vi "AverageAndLog.vi"(5 "error in (no error)":errorcluster) -> (19 "error out":errorcluster)   [LabVIEW 2014, in "IndoorData.lvclass"]
uses:
  IndoorData.lvclass
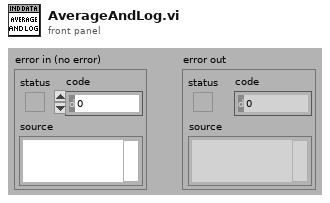
[diagram p1: front panel]
types:
  T1 = enum16{"open", "replace", "create", "open or create", "replace or create", "replace or create with confirmation"}
  T2 = typedef "IndoorData.lvclass/ObjectAttributes.ctl" = cluster{"DebugData":T3, "Actual":T4, "BufferedReadings":T5, "AVGReadings":T5, "LogFolder":path, "FirstLog?":bool, "MinMaxFile":path}
  T3 = typedef "IndoorData.lvclass/DebugData.ctl" = cluster{"Rev":string, "Location":string, "LoopIdx":i32, "PiCoreTemp":dbl, "Error":errorcluster}
  T4 = typedef "IndoorData.lvclass/ActualValues.ctl" = cluster{"Time":dbl, "Temp":dbl, "RH":dbl}
  T5 = typedef "IndoorData.lvclass/BufferedReadings.ctl" = cluster{"Time":dbl[], "Temp":dbl[], "RH":dbl[]}
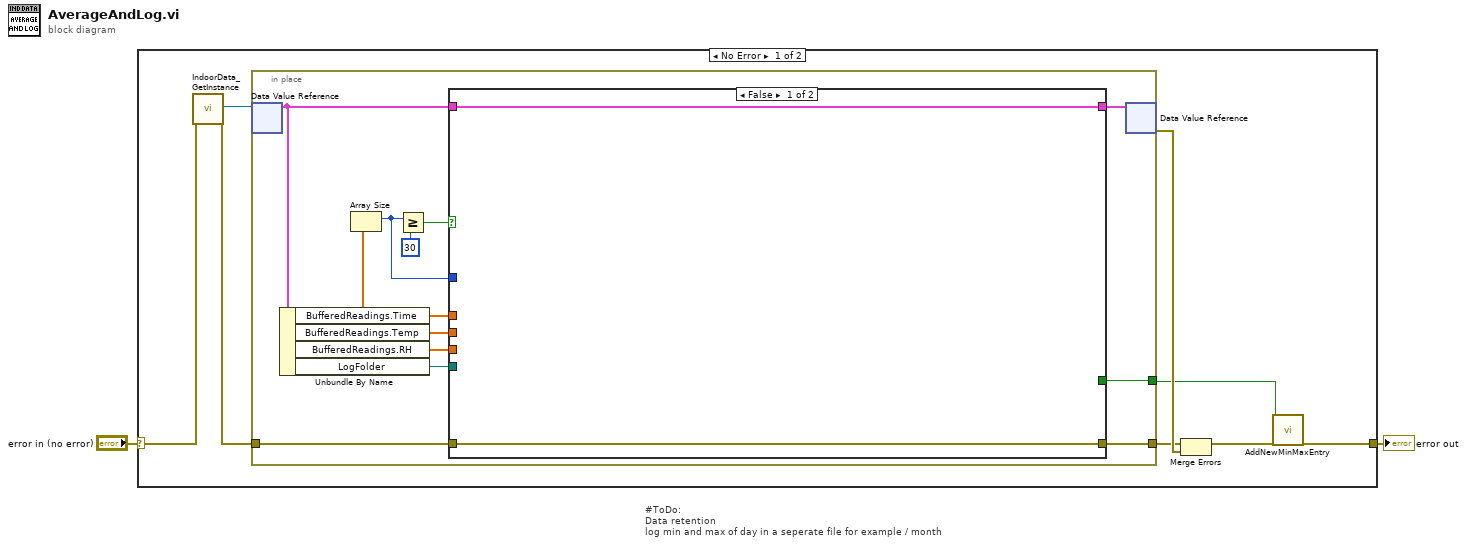
[diagram p0: block diagram]
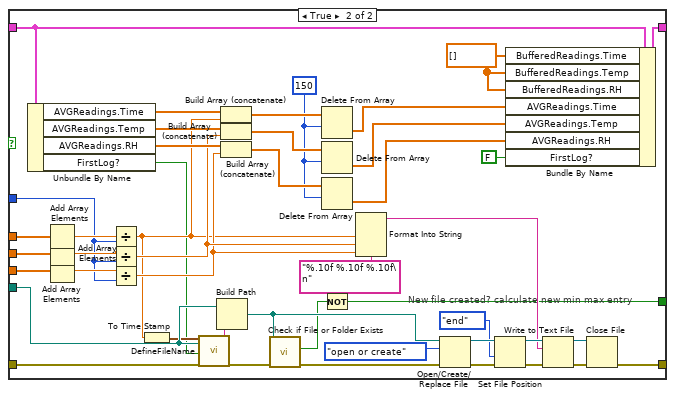
[diagram p2: hidden frame]
diagram:
  # "#ToDo:\nData retention\nlog min and max of day in a seperate file for example / month"
  n1 = case shown="No Error" "error in (no error)" {
    selector: "error in (no error)" -> [w6 w70]
    tunnel: [w4 w70] -> w1
    frame No Error {
      n2 = call "IndoorData_GetInstance.vi"("error in (no error)"=w6) -> ("DVRRefOut"=w9:refnum<data-value>, "error out"=w8:errorcluster)  [unwired: 14 in, 3 out]
      n3 = in-place {
        in-place-border: w8 -> [w17]
        in-place-border: [w18] -> w7
        in-place-border: [w11] -> w3
        n4 = in-place-dvr #1(w9) -> (w21:T2)  [unwired: 1 out]
        n5 = Unbundle By Name(w21) -> ("BufferedReadings.Time"=w16:dbl[], "BufferedReadings.Temp"=w15:dbl[], "BufferedReadings.RH"=w14:dbl[], "LogFolder"=w12:path)
        n6 = Array Size(array=w16) -> (size(s)=w13:i32)
        n7 = Greater Or Equal?(x=w13, y=30) -> (x >= y?=w19:bool)
        n8 = case shown="False" w19 {
          tunnel: [w24 w69] -> w22
          tunnel: w21 -> [w24 w60]
          tunnel: [w23 w37] -> w18
          tunnel: w17 -> [w23 w46]
          tunnel: w16 -> [_ w68]
          tunnel: w15 -> [_ w67]
          tunnel: w14 -> [_ w66]
          tunnel: w13 -> [_ w62]
          tunnel: w12 -> [_ w34]
          tunnel: [_ w25] -> w11
          frame False {
          }
          frame True {
            w53 = 150 ("length")
            w61 = dbl[] [] ("BufferedReadings.Time")
            # "New file created? calculate new min max entry"
            n9 = Unbundle By Name(w60) -> ("AVGReadings.Time"=w59:dbl[], "AVGReadings.Temp"=w58:dbl[], "AVGReadings.RH"=w57:dbl[], "FirstLog?"=w30:bool)
            n10 = Add Array Elements(numeric array=w68) -> (sum=w65:dbl)
            n11 = Add Array Elements(numeric array=w67) -> (sum=w64:dbl)
            n12 = Add Array Elements(numeric array=w66) -> (sum=w63:dbl)
            n13 = Divide(x=w65, y=w62) -> (x/y=w33:dbl)
            n14 = Divide(x=w64, y=w62) -> (x/y=w48:dbl)
            n15 = Divide(x=w63, y=w62) -> (x/y=w47:dbl)
            n16 = To Time Stamp(1:w33) -> (0:w32:timestamp)
            n17 = call "DefineFileName.vi"("Sample Time"=w32, "DataFolder"=w34, "FirstLog?"=w30, "error in (no error)"=w46) -> ("FileName"=w35:string, "error out"=w29:errorcluster)  [unwired: 14 in]
            n18 = Build Path(base path=w34, name or relative path=w35) -> (appended path=w27:path)
            n19 = Build Array (concatenate)(w59, w33) -> (w56:dbl[])
            n20 = Build Array (concatenate)(w58, w48) -> (w55:dbl[])
            n21 = Build Array (concatenate)(w57, w47) -> (w54:dbl[])
            n22 = call <vilib>:"Check if File or Folder Exists.vi"("error in (no error)"=w29, "path"=w27) -> ("error out"=w28:errorcluster, "file or folder exists?"=w26:bool)  [unwired: 7 in, 1 out]
            n23 = Delete From Array(array=w56, length=w53) -> (deleted portion=w50:dbl[])  [unwired: 1 in, 1 out]
            n24 = Delete From Array(array=w55, length=w53) -> (deleted portion=w51:dbl[])  [unwired: 1 in, 1 out]
            n25 = Delete From Array(array=w54, length=w53) -> (deleted portion=w52:dbl[])  [unwired: 1 in, 1 out]
            n26 = Not(x=w26) -> (.not. x?=w25:bool)
            n27 = Format Into String(format string="%.10f %.10f %.10f\n", w33, w48, w47) -> (resulting string=w36:string)  [unwired: 2 in, 1 out]
            n28 = Open/Create/Replace File(file path (use dialog)=w27, error in=w28, operation (0:open)=T1."open or create") -> (refnum out=w44:refnum<file>, error out=w43:errorcluster)  [unwired: 3 in, 1 out]
            n29 = Set File Position(refnum=w44, from (0:start)=enum16{"start", "end", "current"}."end", error in=w43) -> (refnum out=w40:refnum<file>, error out=w41:errorcluster)  [unwired: 1 in]
            n30 = Bundle By Name(cluster=w60, "BufferedReadings.Time"=w61, "BufferedReadings.Temp"=w61, "BufferedReadings.RH"=w61, "AVGReadings.Time"=w50, "AVGReadings.Temp"=w51, "AVGReadings.RH"=w52, "FirstLog?"=FALSE ("Reboot?")) -> (w69:T2)
            n31 = Write to Text File(file (use dialog)=w40, text=w36, error in=w41) -> (refnum out=w39:refnum<file>, error out=w38:errorcluster)  [unwired: 1 in, 1 out]
            n32 = Close File(refnum=w39, error in=w38) -> (error out=w37:errorcluster)  [unwired: 1 out]
          }
        }
        n33 = in-place-dvr #1(w22) -> (w10:errorcluster)  [unwired: 1 out]
      }
      n34 = Merge Errors(w7, w10) -> (w5:errorcluster)
      n35 = call "AddNewMinMaxEntry.vi"("Add New Entry?"=w3, "error in (no error)"=w5) -> ("error out"=w4:errorcluster)  [unwired: 17 in]
    }
    frame Error {
    }
  }
  "error out" <- w1
